vi "SendMessageErrorName.vi"() -> (1 "message name":string)   [LabVIEW 2017, in "ServerComm.lvlib"]
doc: "Returns the following message name: ServerComm.SendMessageError. The NI-developed Server Comm process broadcasts this message when it cannot send a message because the connection between device and server is not online."
uses:
  <vilib>/addons/InsightCM/Devices/Shared/Common/ServerComm/ServerComm.lvlib
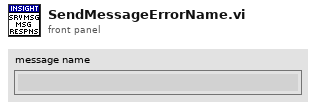
[diagram p1: front panel]
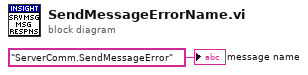
[diagram p0: block diagram]
diagram:
  "message name" <- "ServerComm.SendMessageError" ("ProcessName")
